vi "Power Qualtiy - 6.vi"() -> ()   [LabVIEW 2015]
uses:
  <vilib>/addons/Electrical Power/Power Measurement/subVIs/ep_Filter Design.ctl
  <vilib>/addons/Electrical Power/Power Measurement/NI_EP_Power Measurement.lvlib
panel:
  in  "filter for frequency measurement":T1={"enable filter? (T)"=TRUE, "passband edge frequency [Hz]"=55.0, "passband ripple [dB]"=0.1, "stopband edge frequency [Hz]"=85.0, "stopband attenuation [dB]"=60.0}
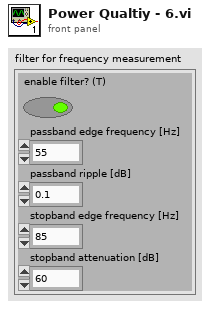
[diagram p1: front panel]
types:
  T1 = typedef "NI_EP_Power Measurement.lvlib/ep_Filter Design.ctl" = cluster{"enable filter? (T)":bool, "passband edge frequency [Hz]":dbl, "passband ripple [dB]":dbl, "stopband edge frequency [Hz]":dbl, "stopband attenuation [dB]":dbl}
  T2 = cluster{"zero crossing times [s]":dbl[], "zero crossings per cycle":u8}
  T3 = typedef "NI_EP_Power Measurement.lvlib/ep_Resampled Data.ctl" = cluster{"times [s]":dbl[], "resampled signal":dbl[]}
  T4 = cluster{"order 0":dbl, "delta order":dbl, "complex spectrum":cdb[]}[]
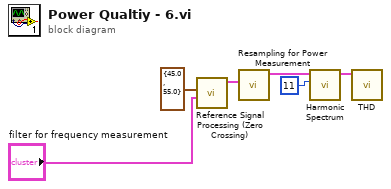
[diagram p0: block diagram]
diagram:
  n1 = call <vilib>:"Reference Signal Processing (Zero Crossing).vi"("filter for frequency measurement"="filter for frequency measurement", "frequency range [Hz]"=cluster{"minimum":dbl, "maximum":dbl} {"minimum"=45.0, "maximum"=55.0}) -> ("zero crossing information"=w6:T2)  [unwired: 6 in, 3 out]
  n2 = call <vilib>:"Resampling for Power Measurement.vi"("trigger information"=w6) -> ("resampled data"=w3:T3[])  [unwired: 9 in, 1 out]
  n3 = call <vilib>:"Harmonic Spectrum.vi"("maximum harmonic order (50)"=u16 11, "resampled data"=w3) -> ("harmonic spectra"=w1:T4)  [unwired: 8 in, 1 out]
  n4 = call <vilib>:"THD.vi"("harmonic spectra"=w1) -> ()  [unwired: 7 in, 4 out]
